vi "imagen_senos_k.vi"(10 "k":dbl, 11 "Image Name":string) -> (3 "Imagen":T1)   [LabVIEW 2020]
uses:
  <vilib>/vision/Image Controls.llb/IMAQ Image.ctl
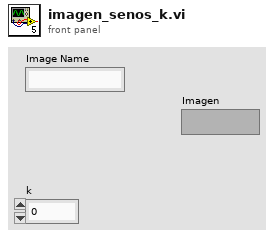
[diagram p1: front panel]
types:
  T1 = typedef "IMAQ Image.ctl" = refnum<image>
  T2 = typedef "Image Type" = u32
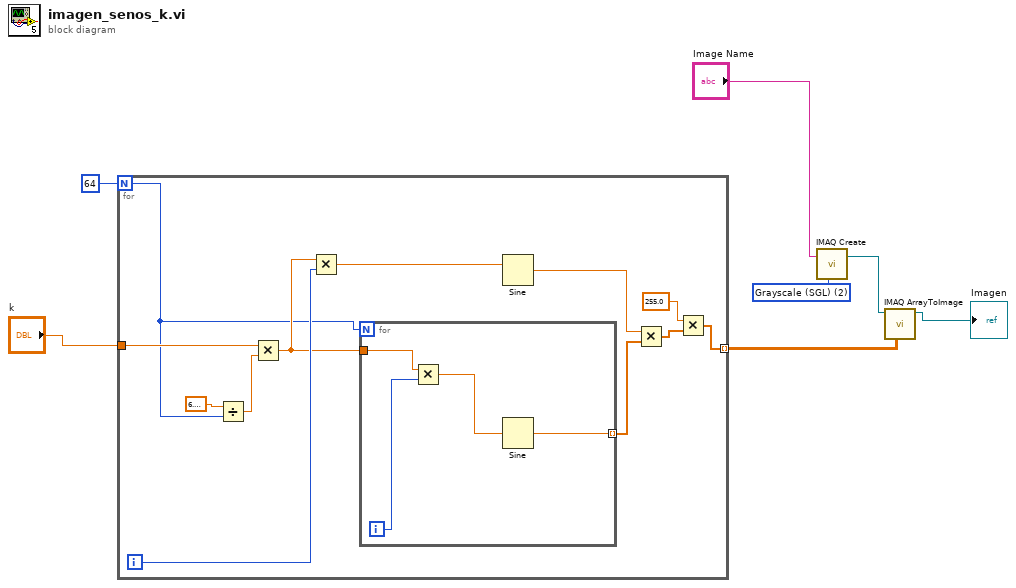
[diagram p0: block diagram]
diagram:
  w3 = T2 2 items=["Grayscale (U8)", "Grayscale (I16)", "Grayscale (SGL)", "Complex (CSG)", "RGB (U32)", "HSL (U32)", "RGB (U64)", "Grayscale (U16)"] ("Image Type")
  n1 = for {
    N: 64 -> [w10]
    tunnel: "k" -> [w12]
    tunnel: [w11] -> w5 mode=indexing
    i -> [w19]
    n2 = Divide(x=6.283185307179586, y=w10) -> (x/y=w9:dbl)
    n3 = Multiply(x=w12, y=w9) -> (x*y=w17:dbl)
    n4 = Multiply(x=w17, y=w19) -> (x*y=w18:dbl)
    n5 = for {
      N: w10 -> [_]
      tunnel: w17 -> [w23]
      tunnel: [w20] -> w15 mode=indexing
      i -> [w22]
      n6 = Multiply(x=w23, y=w22) -> (x*y=w21:dbl)
      n7 = Sine(x=w21) -> (sin(x)=w20:dbl)
    }
    n8 = Sine(x=w18) -> (sin(x)=w16:dbl)
    n9 = Multiply(x=w16, y=w15) -> (x*y=w14:dbl[])
    n10 = Multiply(x=255.0, y=w14) -> (x*y=w11:dbl[])
  }
  n11 = call "IMAQ Create"("Image Name"="Image Name", "Image Type"=w3) -> ("New Image"=w2:T1)  [unwired: 3 in, 1 out]
  n12 = call "IMAQ ArrayToImage"("Image Pixels (Float)"=w5, "Image"=w2) -> ("Image Out"=→"Imagen":T1)  [unwired: 8 in, 1 out]
